vi "FlexDDS-NG_AD9910_FormatSTP.vi"(8 "mirror frequency?":bool, 9 "phase degrees (0..360)":dbl, 10 "amplitude (0..1)":dbl=1.0, 11 "frequency Hz (0..400M)":dbl=10000000.0 format="%^#_6e") -> (0 "phase offset word (POW) out":u16 format="%x", 1 "amplitude scale factor (ASF) out":u16=16383 format="%x", 2 "frequency tuning word (FTW) out":u32=42949673 format="%x", 3 "single-tone profile (STP) out":u64=4611404543493626921 format="%x")   [LabVIEW 2016]
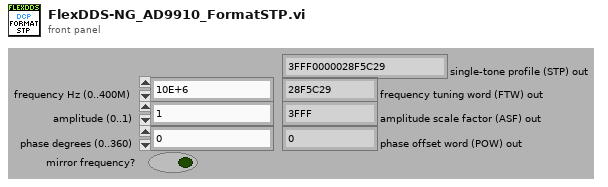
[diagram p1: front panel]
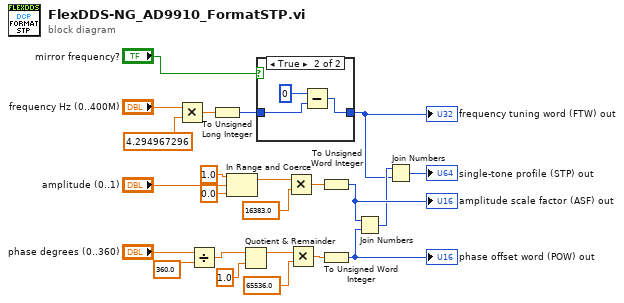
[diagram p0: block diagram]
diagram:
  n1 = Multiply(x="frequency Hz (0..400M)", y=4.294967296) -> (x*y=w13:dbl)
  n2 = Divide(x="phase degrees (0..360)", y=360.0) -> (x/y=w9:dbl)
  n3 = To Unsigned Long Integer(number=w13) -> (unsigned 32bit integer=w7:u32)
  n4 = In Range and Coerce(upper limit=1.0, x="amplitude (0..1)", lower limit=0.0) -> (coerced(x)=w19:dbl)  [unwired: 1 out]
  n5 = Quotient & Remainder(x=w9, y=1.0) -> (x-y*floor(x/y)=w21:dbl)  [unwired: 1 out]
  n6 = case shown="True" "mirror frequency?" {
    tunnel: w7 -> [w24 w26]
    tunnel: [w24 w25] -> w1
    frame False {
    }
    frame True {
      n7 = Subtract(x=u32 0 ("unsigned 32bit integer"), y=w26) -> (x-y=w25:u32)
    }
  }
  "frequency tuning word (FTW) out" <- w1
  n8 = Multiply(x=w19, y=16383.0) -> (x*y=w17:dbl)
  n9 = Multiply(x=w21, y=65536.0) -> (x*y=w16:dbl)
  n10 = To Unsigned Word Integer(number=w17) -> (unsigned 16bit integer=w5:u16)
  "amplitude scale factor (ASF) out" <- w5
  n11 = To Unsigned Word Integer(number=w16) -> (unsigned 16bit integer=w4:u16)
  "phase offset word (POW) out" <- w4
  n12 = Join Numbers(hi=w5, lo=w4) -> ((hi.lo)=w2:u32)
  n13 = Join Numbers(hi=w2, lo=w1) -> ((hi.lo)=→"single-tone profile (STP) out":u64)
